vi "fit function -cos2theta.vi"(3 "output control":T1, 4 "data":T2, 5 "X":dbl[](array[numeric]), 6 "a":dbl[](array[numeric])) -> (0 "error out":errorcluster, 1 "f'(X,a)":dbl[][](array[numeric]), 2 "f(X,a)":dbl[](array[numeric]))   [LabVIEW 2012]
doc: "This template is the starting point for creating a model function to be passed to the Nonlinear Curve Fit.vi."
uses:
  <vilib>/gmath/NumericalOptimization/objective function data.ctl
  <vilib>/gmath/NumericalOptimization/LM_output select.ctl
  <vilib>/gmath/NI_Gmath.lvlib
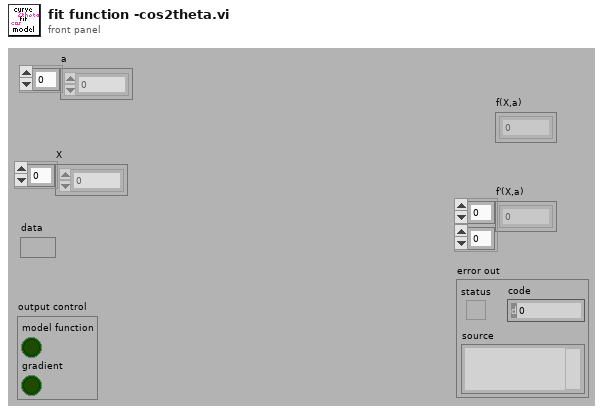
[diagram p1: front panel]
types:
  T1 = typedef "NI_Gmath.lvlib/LM_output select.ctl" = cluster{"model function":bool, "gradient":bool}
  T2 = typedef "NI_Gmath.lvlib/objective function data.ctl" = variant
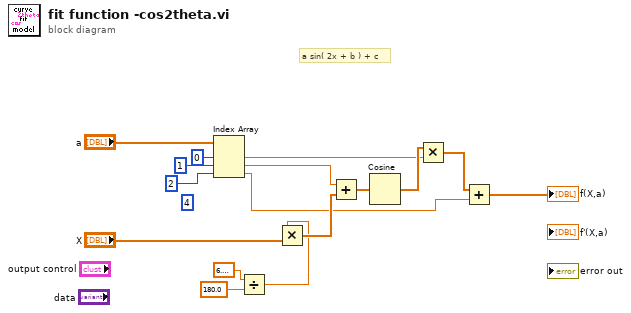
[diagram p0: block diagram]
diagram:
  (unwired) 4 ("index")
  # "a sin( 2x + b ) + c"
  n1 = Index Array(array="a", index #1=0 ("index"), index #2=1 ("index"), index #3=2 ("index")) -> (element #1=w7:dbl, element #2=w2:dbl, element #3=w1:dbl)
  n2 = Divide(x=6.283185307179586, y=180.0) -> (x/y=w3:dbl)
  n3 = Multiply(x=w3, y="X") -> (x*y=w10:dbl[])
  n4 = Add(x=w2, y=w10) -> (x+y=w9:dbl[])
  n5 = Cosine(x=w9) -> (cos(x)=w8:dbl[])
  n6 = Multiply(x=w8, y=w7) -> (x*y=w6:dbl[])
  n7 = Add(x=w6, y=w1) -> (x+y=→"f(X,a)":dbl[])
